vi "WB_convert_to_255_separate_sub_양수.vi"(5 "Weights & Biases":dbl[][](array[numeric])) -> (0 "min value":dbl, 1 "Biases":i64[](array[numeric]), 2 "Weights":i64[][](array[numeric]), 3 "max value":dbl)   [LabVIEW 2021]
panel:
  out "No.Output":i32
  out "No.Input":i32
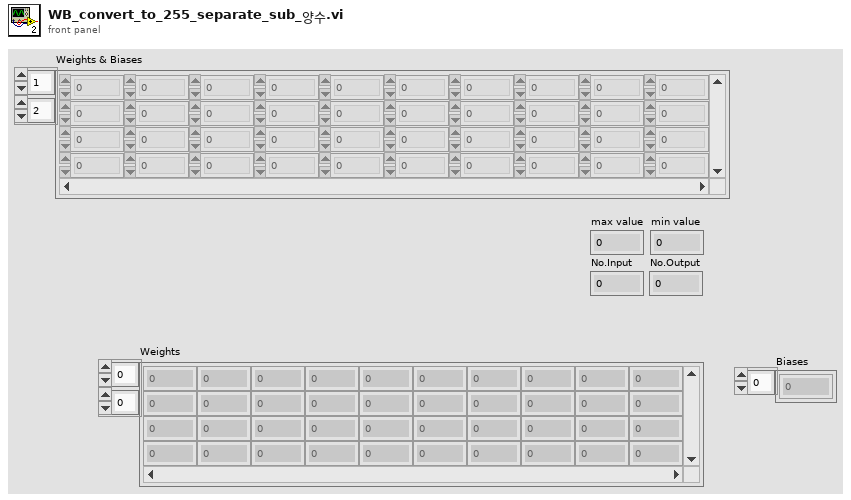
[diagram p1: front panel]
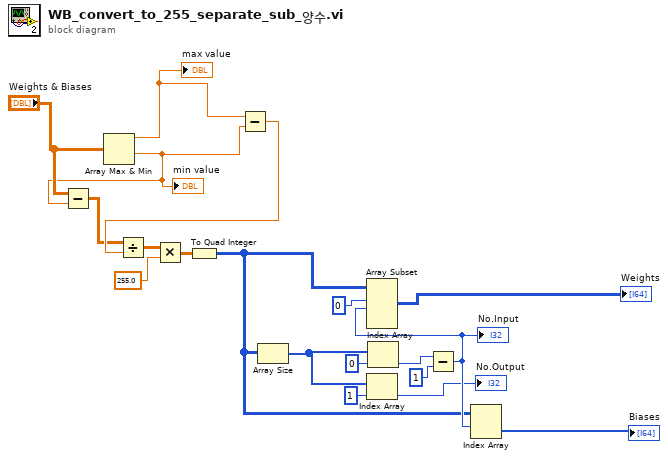
[diagram p0: block diagram]
diagram:
  n1 = Array Max & Min(array="Weights & Biases") -> (max value=w5:dbl, min value=w2:dbl)  [unwired: 2 out]
  "max value" <- w5
  "min value" <- w2
  n2 = Subtract(x="Weights & Biases", y=w2) -> (x-y=w1:dbl[][])
  n3 = Subtract(x=w5, y=w2) -> (x-y=w4:dbl)
  n4 = Divide(x=w1, y=w4) -> (x/y=w8:dbl[][])
  n5 = Multiply(x=w8, y=255.0) -> (x*y=w7:dbl[][])
  n6 = To Quad Integer(1:w7) -> (0:w6:i64[][])
  n7 = Array Size(array=w6) -> (size(s)=w17:i32[])
  n8 = Index Array(array=w17, index=1 ("인덱스")) -> (element=→"No.Output":i32)
  n9 = Index Array(array=w17, index=0 ("인덱스")) -> (element=w15:i32)
  n10 = Subtract(x=w15, y=1) -> (x-y=w13:i32)
  "No.Input" <- w13
  n11 = Array Subset(array=w6, index (row)=0 ("인덱스"), length (row)=w13) -> (→"Weights":i64[][])  [unwired: 2 in]
  n12 = Index Array(array=w6, index (row)=w13) -> (element=→"Biases":i64[])  [unwired: 1 in]
